vi "test -- fucking PID.vi"() -> ()   [LabVIEW 2017]
uses:
  lorentzian.ctl
  circle corners.ctl
  pid -- parameters.ctl
  shake-parameters.ctl
  <vilib>/event_ctls.llb/eventvkey.ctl
  cursor winow.ctl
  agregator -- action.ctl
  cursor window action.ctl
  four-corner circle transformation.ctl
  cursor action.ctl
  linear interpolation - real.vi
  Q -- check range -- i -- real.vi
  draw a line.vi
  draw a circle.vi
  linear interpolation iiii- complex.vi
  Q - not nan -- real.vi
  generate linear region.vi
panel:
  in  "P (sec)":dbl(slide)=0.13219411484660284 scale=0.001..1.0
  in  "I (sec)":dbl(slide)=0.6060606060606061 scale=0.0..3.0
  out "Plot: hist":cluster{"all rows":dbl[], "all rows":dbl[]}[](graph)
  in  "cursor bracket: fit boundaries":T1={"left"=-7.2463869791864255, "right "=9.988059505239747, "center"=1.3708362630266606, "window"=17.234446484426172, "cursors"=[0, 1, 2], "relative"=0, "absolute"=0, "fixed vertical offset"=0.0, "vertical offset"=0.0, "skew"=0.0, "default window frac"=0.1, "kind"=enum."symmetric", "skew.left"=0.5, "skew.right"=0.5, "Plot ref"=refnum, "wing order"=enum."forw"}
  out "Char":i16=50
  out "VKey":T2
  out "center freq (Hz)":dbl=-0.35260838541595674
  out "window  (Hz)":dbl=17.234446484426172
  out "left freq (Hz)":dbl=-8.969831627629043
  out "right freq (Hz)":dbl=8.26461485679713
  in  "dev pars":T3={"base (Hz)"=1000.0, "period(sec)"=20.0, "amp (Hz)"=150.0, "G base (Hz)"=3.0, "G period(sec)"=4.0, "G amp (Hz)"=0.5, "B base (V)"=0.0, "B period(sec)"=40.0, " B amp (V)"=0.1} {"B amp (V)" format="%#_10f"; "B period(sec)" format="%#_10f"; "B base (V)" format="%#_10f"; "G amp (Hz)" format="%#_10f"; "G period(sec)" format="%#_10f"; "G base (Hz)" format="%#_10f"; "amp (Hz)" format="%#_10f"; "period(sec)" format="%#_10f"; "base (Hz)" format="%#_10f"}
  out "time(sec)":dbl=37.07838536100462 format="%#_5f"
  out "off freq":dbl=950.7790087707546 format="%#_5f"
  out "dev frreq":dbl=880.8551992841184 format="%#_5f"
  in  "visc hist time (sec)":dbl=5.0 format="%#_10f"
  in  "PID parameters":T4={"P (sec)"=0.13219411484660284, "I (sec)"=0.6060606060606061}
  out "zi frreq":dbl=1831.634208054873 format="%#_5f"
  out "dev out":cdb=-0.08754535931582605-1.6593232880932235e-06i format="%#_10f"
  out "Plot: complex plane - filter":cluster{dbl[], dbl[]}[](graph)=[{[0.24473620751678493, 0.2444438175497377, 0.24356716059995304, 0.24210777462161087, 0.24006821987361993, 0.2374520744280535, 0.23426392789299527, 0.23050937336080735, 0.2261949975959453, 0.22132836947953544, 0.2159180267309852, 0.20997346092992258, 0.20350510086473944, 0.19652429423695378, 0.18904328775348478, 0.18107520564176743, 0.17263402662539823, 0.16373455940070375, 0.15439241665725545, 0.1446239876879068, 0.13444640963640436, 0.12387753743301488, 0.11293591247090992, 0.10164073007826221, 0.09001180584311719, 0.0780695408501183, 0.06583488589007219, 0.05332930470514255, 0.04057473633415265, 0.027593556624056714, 0.014408538975100763, 0.0010428143885402585, -0.012480169112996431, -0.026136687621306803, -0.03990278296241109, -0.05375430472733049, -0.06766695264011055, -0.08161631918876269, -0.09557793244433395, -0.1095272989929861, -0.12343994690576615, -0.13729146867068548, -0.15105756401178982, -0.16471408252010022, -0.17823706602163691, -0.1916027906081974, -0.20478780825715337, -0.2177689879672493, -0.23052355633823915, -0.24302913752316888, -0.25526379248321496, -0.26720605747621384, -0.2788349817113589, -0.29013016410400666, -0.30107178906611154, -0.311640661269501, -0.32181823932100345, -0.33158666829035216, -0.34092881103380046, -0.34982827825849494, -0.35826945727486414, -0.36623753938658143, -0.3737185458700505, -0.38069935249783615, -0.38716771256301924, -0.39311227836408197, -0.39852262111263215, -0.403389249229042, -0.40770362499390406, -0.41145817952609204, -0.4146463260611502, -0.41726247150671664, -0.41930202625470764, -0.4207614122330498, -0.4216380691828345, -0.4219304591498817, -0.4216380691828345, -0.4207614122330498, -0.41930202625470764, -0.4172624715067167, -0.41464632606115026, -0.4114581795260921, -0.40770362499390417, -0.4033892492290421, -0.3985226211126322, -0.3931122783640821, -0.38716771256301935, -0.38069935249783626, -0.37371854587005066, -0.36623753938658166, -0.3582694572748643, -0.3498282782584951, -0.3409288110338006, -0.3315866682903523, -0.3218182393210036, -0.3116406612695012, -0.30107178906611176, -0.2901301641040068, -0.2788349817113591, -0.26720605747621407, -0.2552637924832152, -0.24302913752316907, -0.23052355633823934, -0.21776898796724944, -0.20478780825715354, -0.19160279060819757, -0.17823706602163697, -0.1647140825201006, -0.1510575640117902, -0.13729146867068587, -0.12343994690576646, -0.10952729899298641, -0.09557793244433425, -0.08161631918876293, -0.06766695264011077, -0.053754304727330726, -0.039902782962411315, -0.026136687621306963, -0.01248016911299657, 0.0010428143885401059, 0.014408538975100693, 0.027593556624056353, 0.04057473633415232, 0.053329304705142216, 0.06583488589007191, 0.07806954085011805, 0.09001180584311694, 0.10164073007826199, 0.11293591247090973, 0.12387753743301472, 0.1344464096364042, 0.14462398768790663, 0.15439241665725534, 0.16373455940070364, 0.17263402662539812, 0.18107520564176738, 0.18904328775348456, 0.19652429423695367, 0.20350510086473933, 0.20997346092992242, 0.2159180267309851, 0.22132836947953533, 0.2261949975959452, 0.2305093733608073, 0.23426392789299527, 0.23745207442805344, 0.24006821987361987, 0.24210777462161087, 0.24356716059995304, 0.2444438175497377], [-0.3333333333333333, -0.31937478209026676, -0.30544071888922814, -0.2915555888118986, -0.27774375109463256, -0.2640294363940802, -0.2504367042783817, -0.23698940101850946, -0.2237111177538056, -0.21062514910510735, -0.1977544523080666, -0.1851216069383575, -0.17274877529942825, -0.16065766354228994, -0.148869483585552, -0.13740491590250895, -0.12628407324056323, -0.11552646533663152, -0.10515096469043711, -0.09517577345573225, -0.08561839150753528, -0.07649558574140364, -0.06782336065860123, -0.05961693028876536, -0.051890691499328345, -0.04465819873852045, -0.03793214025626174, -0.03172431584466018, -0.026045616137166494, -0.02090600350270283, -0.016314494568282156, -0.01227914440078065, -0.008807032375613255, -0.005904249757103797, -0.003575889012337241, -0.0018260348772422552, -0.000657757190576147, -7.310550838485197e-05, -7.310550838485197e-05, -0.000657757190576147, -0.0018260348772421997, -0.003575889012337241, -0.005904249757103741, -0.008807032375613255, -0.012279144400780595, -0.0163144945682821, -0.02090600350270283, -0.02604561613716644, -0.03172431584466012, -0.03793214025626174, -0.04465819873852045, -0.05189069149932829, -0.0596169302887653, -0.06782336065860123, -0.07649558574140353, -0.08561839150753517, -0.09517577345573214, -0.10515096469043705, -0.11552646533663147, -0.12628407324056315, -0.13740491590250892, -0.14886948358555185, -0.16065766354228977, -0.17274877529942811, -0.18512160693835739, -0.19775445230806651, -0.21062514910510727, -0.22371111775380553, -0.2369894010185093, -0.2504367042783816, -0.26402943639408005, -0.27774375109463245, -0.29155558881189847, -0.3054407188892281, -0.3193747820902667, -0.33333333333333315, -0.3472918845763997, -0.3612259477774383, -0.37511107785476794, -0.38892291557203396, -0.40263723027258636, -0.4162299623882848, -0.429677265648157, -0.4429555489128609, -0.45604151756155914, -0.4689122143585999, -0.481545059728309, -0.4939178913672383, -0.5060090031243767, -0.5177971830811146, -0.5292617507641575, -0.5403825934261033, -0.551140201330035, -0.5615157019762295, -0.5714908932109344, -0.5810482751591313, -0.5901710809252629, -0.5988433060080653, -0.6070497363779013, -0.6147759751673383, -0.6220084679281461, -0.6287345264104047, -0.6349423508220065, -0.6406210505295, -0.6457606631639639, -0.6503521720983845, -0.6543875222658859, -0.6578596342910533, -0.6607624169095627, -0.6630907776543293, -0.6648406317894244, -0.6660089094760905, -0.6665935611582818, -0.6665935611582818, -0.6660089094760905, -0.6648406317894244, -0.6630907776543293, -0.6607624169095629, -0.6578596342910534, -0.654387522265886, -0.6503521720983845, -0.6457606631639639, -0.6406210505295002, -0.6349423508220067, -0.628734526410405, -0.6220084679281463, -0.6147759751673385, -0.6070497363779015, -0.5988433060080656, -0.5901710809252632, -0.5810482751591315, -0.5714908932109346, -0.5615157019762296, -0.5511402013300353, -0.5403825934261035, -0.5292617507641577, -0.517797183081115, -0.506009003124377, -0.4939178913672387, -0.4815450597283094, -0.4689122143586003, -0.45604151756155953, -0.44295554891286126, -0.4296772656481574, -0.4162299623882851, -0.4026372302725866, -0.38892291557203423, -0.3751110778547682, -0.3612259477774386, -0.3472918845764]}, {[-0.08859712581654838, -0.08859712581654838, -0.08859712581654838, -0.08859712581654838, -0.08859712581654838, -0.08859712581654838, -0.08859712581654838, -0.08859712581654838, -0.08859712581654838, -0.08859712581654838, -0.08859712581654838, -0.08859712581654838, -0.08859712581654838, -0.08859712581654838, -0.08859712581654838, -0.08859712581654838, -0.08859712581654838, -0.08859712581654838, -0.08859712581654838, -0.08859712581654838], [0.0, -0.03333333333333333, -0.06666666666666667, -0.1, -0.13333333333333333, -0.16666666666666666, -0.2, -0.23333333333333334, -0.26666666666666666, -0.3, -0.3333333333333333, -0.36666666666666664, -0.4, -0.43333333333333335, -0.4666666666666667, -0.5, -0.5333333333333333, -0.5666666666666667, -0.6, -0.6333333333333333]}, {[0.24473620751678493, 0.2114028741834516, 0.17806954085011828, 0.14473620751678493, 0.1114028741834516, 0.07806954085011827, 0.04473620751678492, 0.011402874183451595, -0.02193045914988173, -0.05526379248321506, -0.08859712581654838, -0.12193045914988171, -0.1552637924832151, -0.18859712581654842, -0.22193045914988174, -0.25526379248321507, -0.2885971258165484, -0.3219304591498817, -0.35526379248321505, -0.38859712581654837], [-0.3333333333333333, -0.3333333333333333, -0.3333333333333333, -0.3333333333333333, -0.3333333333333333, -0.3333333333333333, -0.3333333333333333, -0.3333333333333333, -0.3333333333333333, -0.3333333333333333, -0.3333333333333333, -0.3333333333333333, -0.3333333333333333, -0.3333333333333333, -0.3333333333333333, -0.3333333333333333, -0.3333333333333333, -0.3333333333333333, -0.3333333333333333, -0.3333333333333333]}]
  out "Plot: circle sweep window":cluster{dbl[], dbl[]}[](graph)
  out "dt (sec)":dbl=0.004 format="%#_10f"
  in  "total number of point":dbl=50000.0 format="%#_10f"
  in  "total exp time (sec)":dbl=200.0 format="%#_10f"
  in  "zi frequency (Hz)":dbl=1000.0 format="%#_10f"
  in  "lorentzian -- basic":T5={"Amplitude"=1.0, "omega(0)"=1000.0, "Gamma"=3.0, "phase"=0.0, "Q"=300.0, "Norm  Ampl"=nan, "z (inf)"=0.0+0.0i, "4corners"={"z (-pi/2)"=9.277908004825974e-07+0.0007240755403629966i, "z(inf)"=2.6527949823343002e-05+0.0007477540585896028i, "z (pi/2)"=2.8494315967368497e-06+0.0007733542176124632i, "z center"=1.8886111986097237e-06+0.0007487148789877299i, "z(0)"=-2.2750727426123552e-05+0.000749675699385857i, "radius"=2.4658065287076567e-05}} {"z (inf)" format="%#9_9f"; "Q" format="%#9_9f"; "phase" format="%#9_9f"; "Gamma" format="%#9_9f"; "omega(0)" format="%#9_9f"}
  # "Gamma"
  # "backgr"
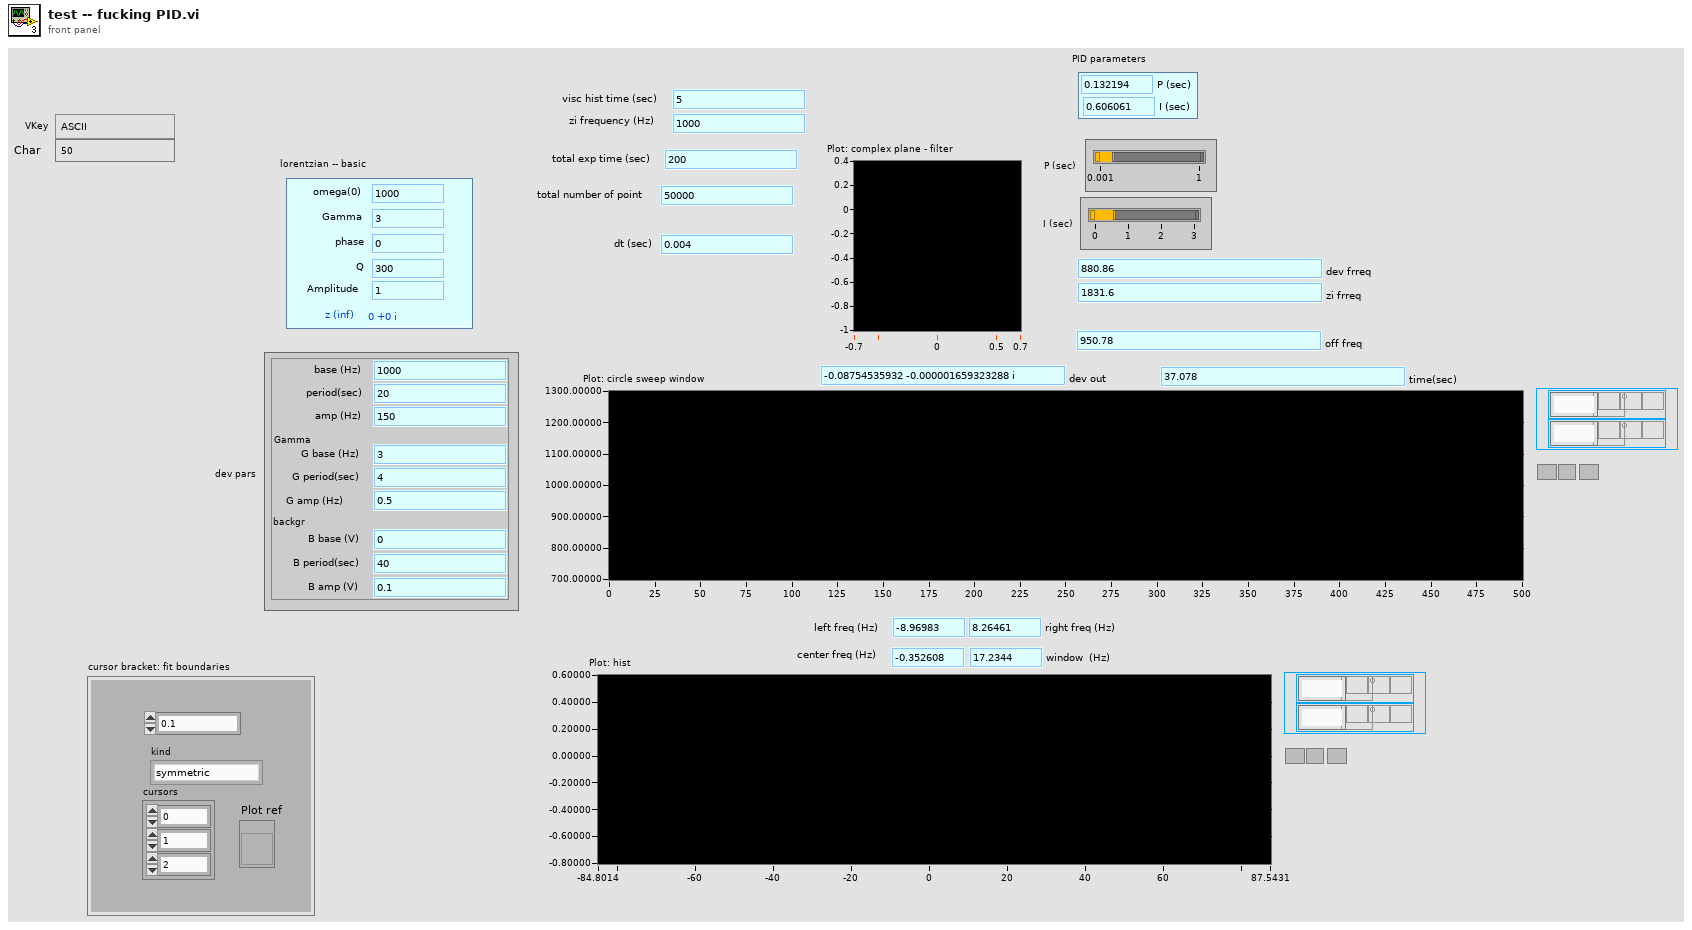
[diagram p1: front panel]
types:
  T1 = typedef "cursor winow.ctl" = cluster{"left":dbl, "right ":dbl, "center":dbl, "window":dbl, "cursors":i32[], "relative":i32, "absolute":i32, "fixed vertical offset":dbl, "vertical offset":dbl, "skew":dbl, "default window frac":dbl, "kind":enum16{"symmetric", "skewed", "fancy"}, "skew.left":dbl, "skew.right":dbl, "Plot ref":refnum<vi>, "wing order":enum16{"forw", "back"}}
  T2 = typedef "eventvkey.ctl" = enum16{"ASCII", "Enter", "Return", "Shift", "Ctrl", "Alt", "Cmd", "Opt", "Caps", "NumLock", "Clear", "Break", "Up", "Down", "Left", "Right", "Insert", "Delete", "Home", "End", "PageUp", "PageDown", "Escape", "Help", "Pause", "ScrollLock", "F1", "F2", "F3", "F4", "F5", "F6", "F7", "F8", "F9", "F10", "F11", "F12", "F13", "F14", "F15", "F16", "F17", "F18", "F19", "F20", "F21", "F22", "F23", "F24", "Play", "VolumeUp", "VolumeDown", "Mute", "Two Byte Char"}
  T3 = typedef "shake-parameters.ctl" = cluster{"base (Hz)":dbl, "period(sec)":dbl, "amp (Hz)":dbl, "G base (Hz)":dbl, "G period(sec)":dbl, "G amp (Hz)":dbl, "B base (V)":dbl, "B period(sec)":dbl, " B amp (V)":dbl}
  T4 = typedef "pid -- parameters.ctl" = cluster{"P (sec)":dbl, "I (sec)":dbl}
  T5 = typedef "lorentzian.ctl" = cluster{"Amplitude":dbl, "omega(0)":dbl, "Gamma":dbl, "phase":dbl, "Q":dbl, "Norm  Ampl":dbl, "z (inf)":cdb, "4corners":T6}
  T6 = typedef "circle corners.ctl" = cluster{"z (-pi/2)":cdb, "z(inf)":cdb, "z (pi/2)":cdb, "z center":cdb, "z(0)":cdb, "radius":dbl}
  T7 = typedef "cursor window action.ctl" = enum16{"balance", "h. offset change", "cursor moves", "change center", "change window", "init", "check", "reset", "set y to middle", "idle", "-write all Y", "-write left.X", "-write center.X", "-write right.X", "-write all X", "-change center", "-change window", "-change skew", "-read cursor 2", "-read cursor 1", "-read cursor 0", "-read all cursors", "-reset", "-read plot scale", "-set y to middle", "-Q: center.Y is visible", "-Q: window is visible", "-parse center.Y", "-right left from center", "-left move", "-right move", "-set center.Y", "-empty", "-set cursors to default", "-check", "-write center.Y", "-copy cursor 1", "-copy cursor 0", "-copy cursor 2", "move right", "move left", "shrink", "broaden", "skew up", "skew down", "-write plot scale", "zoom X", "change cen&win", "zoom to all data", "color--red", "color--green", "color--yellow", "read", "zoom out", "zoom in", "slide right", "slide left"}
  T8 = typedef "agregator -- action.ctl" = enum16{"append", "interpolate", "empty!", "force", "init", "scale", "read last"}
  T9 = typedef "cursor action.ctl" = enum16{"range", "read", "write", "check", "zoom out", "smart zoom out"}
  T10 = typedef "four-corner circle transformation.ctl" = enum16{"z(c) z(inf)", "z(c) z(zero)", "fix phase", "calculate lorentzian", "z(0) z(+-pi/2)", "shift to zcenter", "to  canonical", "get canonical phase", "get4corners"}
  T11 = typedef "interpolation state - complex.ctl" = cluster{"requested size":i32, "Array":cdb[], "actual number of elements":i32}
  T12 = typedef "interpolation state - real.ctl" = cluster{"requested size":i32, "Array":dbl[], "actual number of elements":i32}
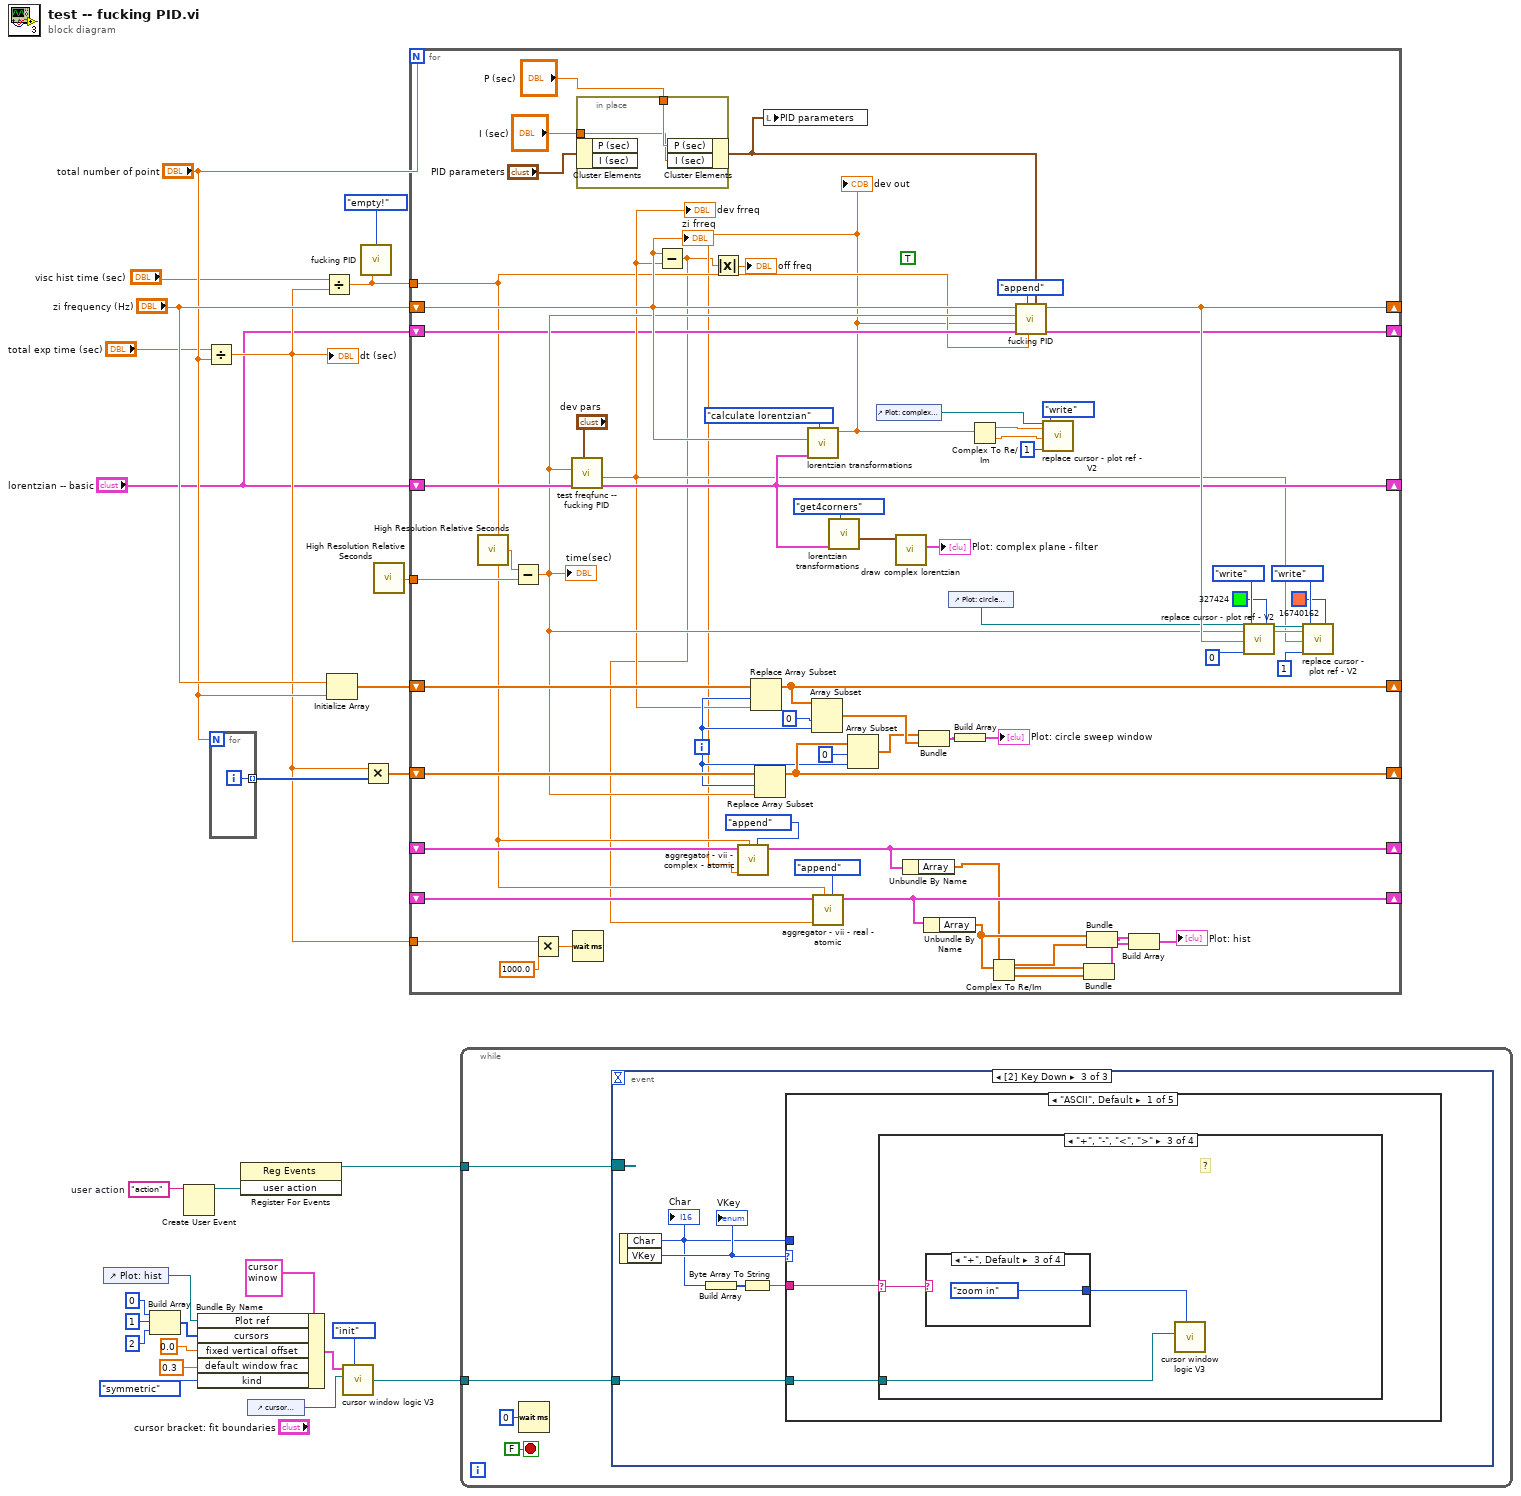
[diagram p0: block diagram]
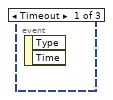
[diagram p2: hidden frame]
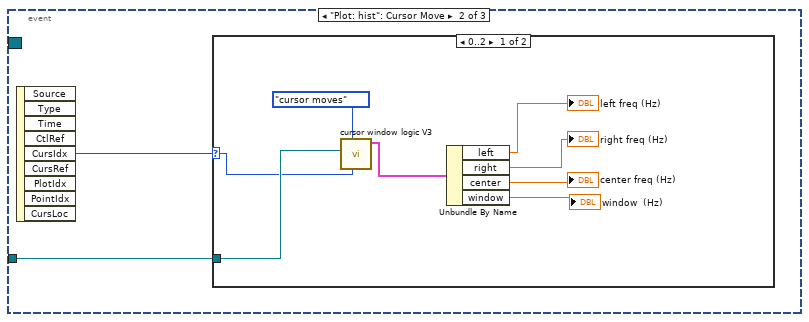
[diagram p3: hidden frame]
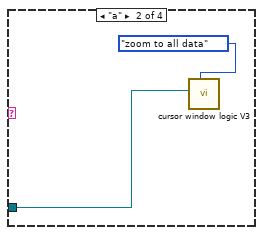
[diagram p6: hidden frame]
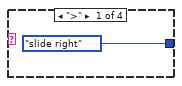
[diagram p7: hidden frame]
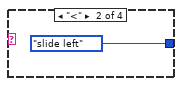
[diagram p8: hidden frame]
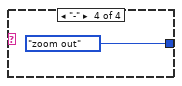
[diagram p9: hidden frame]
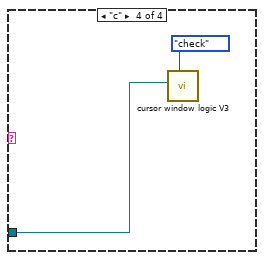
[diagram p10: hidden frame]
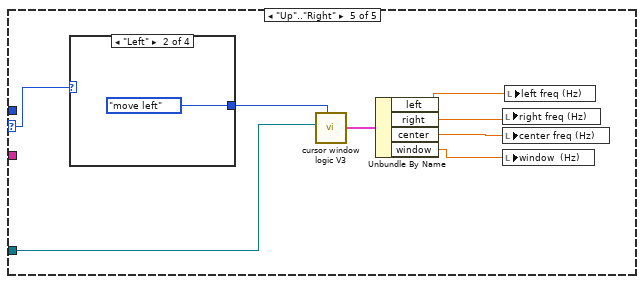
[diagram p14: hidden frame]
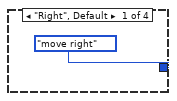
[diagram p15: hidden frame]
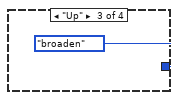
[diagram p16: hidden frame]
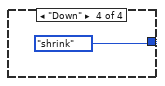
[diagram p17: hidden frame]
diagram:
  w14 = "action"  # user action
  n1 = control-ref of="Plot: hist"() -> (w12:refnum<vi>)
  n2 = Build Array(0, 1, 2) -> (w1:i32[])
  n3 = Create User Event(user event datatype=w14) -> (user event=w15:refnum<user-event>)  [unwired: 1 in, 1 out]
  n4 = Bundle By Name(cluster=T1 {"left"=0.0, "right "=0.0, "center"=0.0, "window"=0.0, "cursors"=[], "relative"=0, "absolute"=0, "fixed vertical offset"=0.0, "vertical offset"=0.0, "skew"=0.0, "default window frac"=0.0, "kind"=enum."symmetric", "skew.left"=0.0, "skew.right"=0.0, "Plot ref"=refnum, "wing order"=enum."forw"} ("cursor bracket: All, data window"), "Plot ref"=w12, "cursors"=w1, "fixed vertical offset"=0.0, "default window frac"=0.3 ("fixed vertical offset"), "kind"=enum16{"symmetric", "skewed", "fancy"}."symmetric") -> (w9:T1)
  n5 = Divide(x="total exp time (sec)", y="total number of point") -> (x/y=w21:dbl)
  "dt (sec)" <- w21
  n6 = for {
    N: "total number of point" -> [_]
    tunnel: [w29] -> w23 mode=indexing
    i -> [w29]
  }
  n7 = register-events(w15) -> (reference out=w13:refnum<event-registration>)  [unwired: 2 in, 1 out]
  n8 = control-ref of="cursor bracket: fit boundaries"() -> (w11:refnum<vi>)
  n9 = Divide(x="visc hist time (sec)", y=w21) -> (x/y=w18:dbl)
  n10 = Initialize Array("zi frequency (Hz)", "total number of point") -> (w26:dbl[])
  n11 = call "cursor window logic V3.vi"("cursor window action"=cursor_window_action."init", "cursor window in"=w11, "cursor window init"=w9) -> ("cursor window out"=w16:refnum<vi>)  [unwired: 7 in, 1 out]
  n12 = call "fucking PID.vi"("requested size"=w18, "PID action"=agregator_--_action."empty!") -> ()  [unwired: 6 in, 4 out]
  n13 = Multiply(x=w21, y=w23) -> (x*y=w22:dbl[])
  n14 = call <vilib>:"High Resolution Relative Seconds.vi"() -> ("relative seconds"=w28:dbl)
  n15 = for {
    N: "total number of point" -> [_]
    shift-right: [w77] -> _
    shift-left: "zi frequency (Hz)" -> [w62]
    shift-right: [w59] -> _
    shift-left: "lorentzian -- basic" -> [w60]
    tunnel: w28 -> [w93]
    shift-right: [w69] -> _
    shift-left: w26 -> [w92]
    shift-right: [w65] -> _
    shift-left: w22 -> [w91]
    tunnel: w21 -> [w88]
    tunnel: w18 -> [w42]
    shift-right: [w54] -> _
    shift-left: "lorentzian -- basic" -> [w53]
    shift-right: [w37] -> _
    shift-left: _ -> [w46]
    shift-right: [w39] -> _
    shift-left: _ -> [w43]
    i -> [w63]
    (unwired) TRUE
    n16 = call <vilib>:"High Resolution Relative Seconds.vi"() -> ("relative seconds"=w90:dbl)
    n17 = Subtract(x=w90, y=w93) -> (x-y=w58:dbl)
    "time(sec)" <- w58
    n18 = Multiply(x=w88, y=1000.0) -> (x*y=w89:dbl)
    n19 = call "test freqfunc -- fucking PID.vi"("pars"="dev pars", "lorentzian -- basic"=w60, "time (sec)"=w58) -> ("lorentzian -- basic -- OUT"=w59:T5, "freq (Hz)"=w57:dbl)  [unwired: 7 in]
    "dev frreq" <- w57
    n20 = Wait (ms)(milliseconds to wait=w89) -> ()  [unwired: 1 out]
    n21 = in-place {
      in-place-border: "P (sec)" -> [w95]
      in-place-border: "I (sec)" -> [w94]
      n22 = in-place-cluster #1("PID parameters") -> ()  [unwired: 2 out]
      n23 = in-place-cluster #1("P (sec)"=w95, "I (sec)"=w94) -> (w30:T4)
    }
    n24 = Subtract(x=w62, y=w57) -> (x-y=w35:dbl)
    n25 = Absolute Value(x=w35) -> (abs(x)=→"off freq":dbl)
    n26 = Replace Array Subset(array=w92, new element=w57, index=w63) -> (w69:dbl[])
    n27 = Replace Array Subset(array=w91, new element=w58, index=w63) -> (w65:dbl[])
    n28 = local write "PID parameters"(w30) -> ()
    n29 = call "lorentzian transformations.vi"("4 corner circle transformation"=four-corner_circle_transformation."calculate lorentzian", "lorentzian in"=w59, "freq in"=w62) -> ("voltage out"=w40:cdb)  [unwired: 6 in, 2 out]
    "dev out" <- w40
    n30 = call "aggregator - vii - complex - atomic.vi"("aggregator action"=agregator_--_action."append", "requested size"=w42, "number"=w40, "state IN"=w46) -> ("state OUT"=w37:T11)  [unwired: 4 in, 3 out]
    n31 = Array Subset(array=w69, index=0 ("cursor index"), length=w63) -> (w67:dbl[])
    n32 = call "aggregator - vii - real - atomic.vi"("aggregator action"=agregator_--_action."append", "requested size"=w42, "number"=w35, "state IN"=w43) -> ("state OUT"=w39:T12)  [unwired: 4 in, 3 out]
    n33 = call "lorentzian transformations.vi"("4 corner circle transformation"=four-corner_circle_transformation."get4corners", "lorentzian in"=w59) -> ("4corners our"=w85:T6)  [unwired: 7 in, 2 out]
    n34 = Array Subset(array=w65, index=0 ("cursor index"), length=w63) -> (w66:dbl[])
    n35 = control-ref of="Plot: complex plane - filter"() -> (w78:refnum<vi>)
    n36 = call "draw complex lorentzian.vi"("4 corners"=w85) -> ("fancy circles"=→"Plot: complex plane - filter":cluster{dbl[], dbl[]}[])  [unwired: 10 in]
    n37 = Unbundle By Name(w37) -> ("Array"=w36:cdb[])
    n38 = Bundle(w66, w67) -> (w75:cluster{dbl[], dbl[]})  [unwired: 1 in]
    n39 = Unbundle By Name(w39) -> ("Array"=w38:dbl[])
    n40 = control-ref of="Plot: circle sweep window"() -> (w70:refnum<vi>)
    n41 = Build Array(w75) -> (→"Plot: circle sweep window":cluster{dbl[], dbl[]}[])
    n42 = Complex To Re/Im(x + iy=w40) -> (x=w80:dbl, y=w79:dbl)
    n43 = Complex To Re/Im(x + iy=w36) -> (x=w51:dbl[], y=w50:dbl[])
    n44 = call "fucking PID.vi"("PID parameters"=w30, "requested size"=w42, "PID action"=agregator_--_action."append", "lorentzian IN"=w53, "voltage IN (V)"=w40, "time in (sec)"=w58, "frequency IN (Hz)"=w62) -> ("lorentzian  OUT"=w54:T5, "frequency out (Hz)"=w77:dbl)  [unwired: 1 in, 2 out]
    n45 = call "replace cursor - plot ref - V2.vi"("Plot ref in"=w78, "new X"=w80, "new  Y"=w79, "cursor index"=1, "cursor action"=cursor_action."write") -> ()  [unwired: 12 in, 3 out]
    n46 = Bundle("Array"=w38, w50) -> (w48:cluster{"Array":dbl[], dbl[]})  [unwired: 1 in]
    n47 = Bundle("Array"=w38, w51) -> (w49:cluster{"Array":dbl[], dbl[]})  [unwired: 1 in]
    n48 = Build Array(w49, w48) -> (→"Plot: hist":cluster{"Array":dbl[], dbl[]}[])
    n49 = call "replace cursor - plot ref - V2.vi"("Plot ref in"=w70, "new X"=w58, "new  Y"=w77, "cursor index"=0, "cursor action"=cursor_action."write", "Color Box"=u32 327424) -> ("Plot ref out"=w61:refnum<vi>)  [unwired: 11 in, 2 out]
    n50 = call "replace cursor - plot ref - V2.vi"("Plot ref in"=w61, "new X"=w58, "new  Y"=w57, "cursor index"=1, "cursor action"=cursor_action."write", "Color Box"=u32 16740162) -> ()  [unwired: 11 in, 3 out]
    "zi frreq" <- w62
  }
  n51 = while {
    tunnel: w13 -> [w99]
    tunnel: w16 -> [w97]
    stop <- FALSE stop-if-true
    n52 = Wait (ms)(milliseconds to wait=u32 0) -> ()  [unwired: 1 out]
    n53 = event shown="[2] Key Down" {
      selector: w99 -> [_ _ _]
      dyn-events: _ -> [_ _ _]
      timeout: _ -> [_ _ _]
      tunnel: w97 -> [_ w101 w110]
      event Timeout {
        n54 = event-data() -> ()  [unwired: 1 in, 2 out]
      }
      event "Plot: hist": Cursor Move {
        n55 = event-data() -> ("CursIdx"=w100:i32)  [unwired: 1 in, 8 out]
        n56 = case shown="0..2" w100 {
          selector: w100 -> [w107 _]
          tunnel: w101 -> [w109 _]
          frame 0..2 {
            n57 = call "cursor window logic V3.vi"("CursIdx"=w107, "cursor window action"=cursor_window_action."cursor moves", "cursor window in"=w109) -> ("cursor window out"=w106:T1)  [unwired: 7 in, 1 out]
            n58 = Unbundle By Name(w106) -> ("left"=→"left freq (Hz)":dbl, "right"=→"right freq (Hz)":dbl, "center"=→"center freq (Hz)":dbl, "window"=→"window  (Hz)":dbl)
          }
          frame 3, Default {
          }
        }
      }
      event Key Down {
        n59 = event-data() -> ("Char"=w112:i16, "VKey"=w114:T2)  [unwired: 1 in]
        "Char" <- w112
        "VKey" <- w114
        n60 = Build Array(w112) -> (w113:i16[])
        n61 = Byte Array To String(unsigned byte array=w113) -> (string=w111:string)
        n62 = case shown="\"ASCII\", Default" w114 {
          selector: w114 -> [_ _ _ _ w135]
          tunnel: w112 -> [_ _ _ _ _]
          tunnel: w111 -> [w116 _ _ _ _]
          tunnel: w110 -> [w115 _ _ _ w128]
          frame "ASCII", Default {
            n63 = case shown="\"+\", \"-\", \"<\", \">\"" w116 {
              selector: w116 -> [_ _ w120 _]
              tunnel: w115 -> [_ w117 w121 w126]
              frame "0", Default {
              }
              frame "a" {
                n64 = call "cursor window logic V3.vi"("cursor window action"=cursor_window_action."zoom to all data", "cursor window in"=w117) -> ()  [unwired: 8 in, 2 out]
              }
              frame "+", "-", "<", ">" {
                # "?"
                n65 = case shown="\"+\", Default" w120 {
                  tunnel: [cursor_window_action."slide right" ("cursor window action") cursor_window_action."slide left" ("cursor window action") cursor_window_action."zoom in" ("cursor window action") cursor_window_action."zoom out" ("cursor window action")] -> w119
                  frame ">" {
                  }
                  frame "<" {
                  }
                  frame "+", Default {
                  }
                  frame "-" {
                  }
                }
                n66 = call "cursor window logic V3.vi"("cursor window action"=w119, "cursor window in"=w121) -> ()  [unwired: 8 in, 2 out]
              }
              frame "c" {
                n67 = call "cursor window logic V3.vi"("cursor window action"=cursor_window_action."check", "cursor window in"=w126) -> ()  [unwired: 8 in, 2 out]
              }
            }
          }
          frame "Escape" {
          }
          frame "PageUp" {
          }
          frame "PageDown" {
          }
          frame "Up".."Right" {
            n68 = case shown="\"Left\"" w135 {
              tunnel: [cursor_window_action."move right" ("cursor window action") cursor_window_action."move left" ("cursor window action") cursor_window_action."broaden" ("cursor window action") cursor_window_action."shrink" ("cursor window action")] -> w130
              frame "Right", Default {
              }
              frame "Left" {
              }
              frame "Up" {
              }
              frame "Down" {
              }
            }
            n69 = call "cursor window logic V3.vi"("cursor window action"=w130, "cursor window in"=w128) -> ("cursor window out"=w129:T1)  [unwired: 8 in, 1 out]
            n70 = Unbundle By Name(w129) -> ("left"=w134:dbl, "right"=w133:dbl, "center"=w132:dbl, "window"=w131:dbl)
            n71 = local write "right freq (Hz)"(w133) -> ()
            n72 = local write "center freq (Hz)"(w132) -> ()
            n73 = local write "window  (Hz)"(w131) -> ()
            n74 = local write "left freq (Hz)"(w134) -> ()
          }
        }
      }
    }
  }
